vi "RemoteConf.vi"(7 "Write?":bool, 11 "ConfInput":T1={"1B1-12:2B1-12:1POV:2POV"=[TRUE, TRUE, TRUE, TRUE, TRUE, TRUE, TRUE, TRUE, TRUE, TRUE, TRUE, TRUE, TRUE, TRUE, TRUE, TRUE, TRUE, TRUE, TRUE, TRUE, TRUE, TRUE, TRUE, TRUE, TRUE, TRUE], "1LXY:RXY:2LXY:RXY"=[TRUE, TRUE, TRUE, TRUE, TRUE, TRUE, TRUE, TRUE]}) -> (3 "Conf":T1={"1B1-12:2B1-12:1POV:2POV"=[TRUE, TRUE, TRUE, TRUE, TRUE, TRUE, TRUE, TRUE, TRUE, TRUE, TRUE, TRUE, TRUE, TRUE, TRUE, TRUE, TRUE, TRUE, TRUE, TRUE, TRUE, TRUE, TRUE, TRUE, TRUE, TRUE], "1LXY:RXY:2LXY:RXY"=[TRUE, TRUE, TRUE, TRUE, TRUE, TRUE, TRUE, TRUE]})   [LabVIEW 2010, in "Packet Recorder.lvlib"]
uses:
  Packet Recorder.lvlib
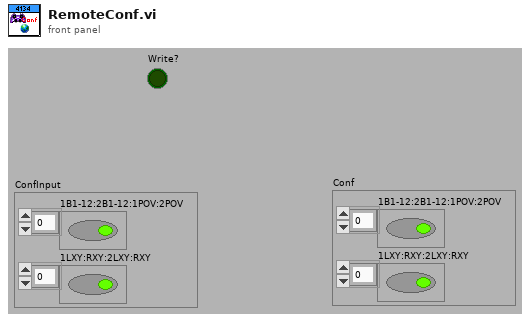
[diagram p1: front panel]
types:
  T1 = cluster{"1B1-12:2B1-12:1POV:2POV":bool[], "1LXY:RXY:2LXY:RXY":bool[]}
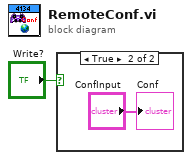
[diagram p0: block diagram]
diagram:
  n1 = case shown="True" "Write?" {
    frame False {
    }
    frame True {
      "Conf" <- "ConfInput"
    }
  }
